vi "Send Message and Wait for Response.vi"(6 "Timeout":i32=1000, 7 "Message Priority (Normal)":T1=enum."Normal", 8 "error in":errorcluster, 9 "DataSocket Reply URL":string, 10 "Original Message":refnum<class "Reply Msg DataSocket.lvclass">, 11 "Message Enqueuer in":refnum<class "Message Enqueuer.lvclass">) -> (0 "error out":errorcluster, 1 "Timeout?":bool, 2 "Reply":variant, 3 "Message Enqueuer out":refnum<class "Message Enqueuer.lvclass">)   [LabVIEW 2023, in "Reply Msg DataSocket.lvclass"]
uses:
  Reply Msg DataSocket.lvclass
  <vilib>/ActorFramework/Message Enqueuer/Message Enqueuer.lvclass
  <vilib>/ActorFramework/Message Enqueuer/Message Priority.ctl
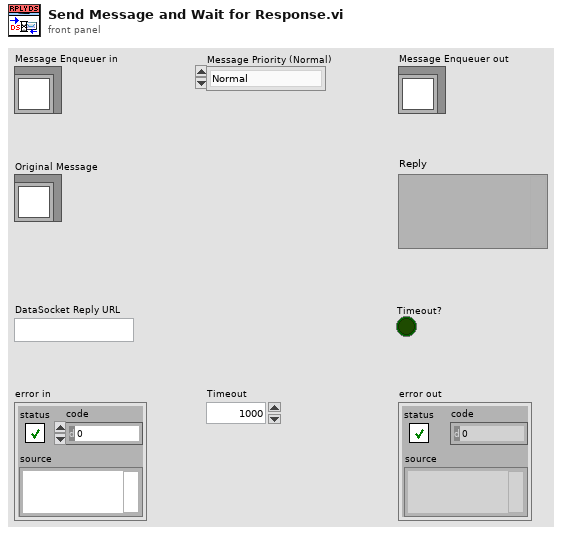
[diagram p1: front panel]
types:
  T1 = typedef "Actor Framework.lvlib/Message Enqueuer.lvclass/Message Priority.ctl" = enum16{"Low", "Normal", "High"}
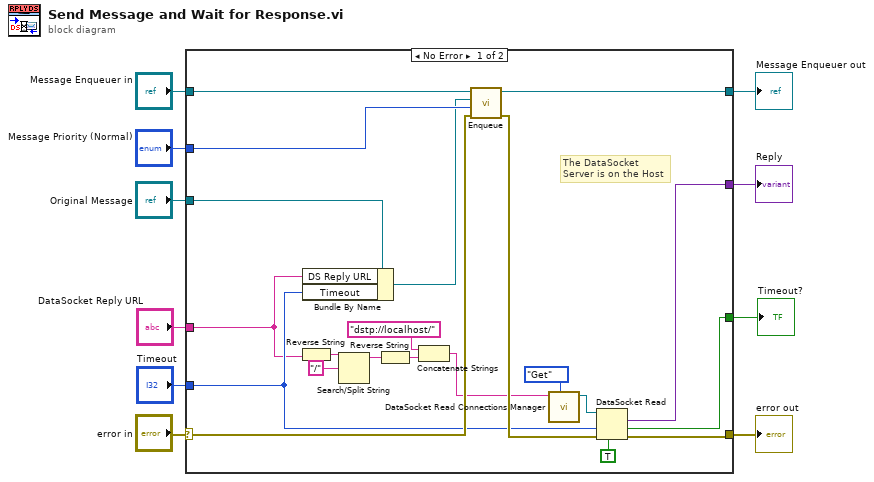
[diagram p0: block diagram]
diagram:
  n1 = case shown="No Error" "error in" {
    selector: "error in" -> [w28 w33]
    tunnel: [w24 w33] -> w5
    tunnel: "Original Message" -> [w27 _]
    tunnel: "Message Enqueuer in" -> [w31 w32]
    tunnel: [w22 _] -> w8
    tunnel: "Message Priority (Normal)" -> [w30 _]
    tunnel: [w29 w32] -> w7
    tunnel: [w23 _] -> w3
    tunnel: "Timeout" -> [w20 _]
    tunnel: "DataSocket Reply URL" -> [w19 _]
    frame No Error {
      # "The DataSocket\nServer is on the Host"
      n2 = Reverse String(1:w19) -> (0:w18:string)
      n3 = Bundle By Name(cluster=w27, "DS Reply URL"=w19, "Timeout"=w20) -> (w26:refnum<class "Reply Msg DataSocket.lvclass">)
      n4 = Search/Split String(string=w18, search string/char (-)="/") -> (substring before match=w14:string)  [unwired: 1 in, 2 out]
      n5 = Reverse String(1:w14) -> (0:w15:string)
      n6 = Concatenate Strings("dstp://localhost/" ("string"), w15) -> (w11:string)
      n7 = call <vilib>:"Enqueue.vi"("error in (no error)"=w28, "Message Priority (Normal)"=w30, "Message"=w26, "Message Enqueuer in"=w31) -> ("error out"=w25:errorcluster, "Message Enqueuer out"=w29:refnum<class "Message Enqueuer.lvclass">)  [unwired: 6 in]
      n8 = call "DataSocket Read Connections Manager.vi"("Action"=enum16{"Get", "Close", "Close All"}."Get", "URL"=w11) -> ("connection id"=w13:refnum<k13>)  [unwired: 9 in]
      n9 = DataSocket Read(6:TRUE ("wait for updated value (T)"), 8:w25, 9:w20, 11:w13) -> (0:w24:errorcluster, 1:w23:bool, 2:w22:variant)  [unwired: 1 in, 4 out]
    }
    frame Error {
    }
  }
  "error out" <- w5
  "Reply" <- w8
  "Message Enqueuer out" <- w7
  "Timeout?" <- w3
